vi "Package Name.vi"(8 "error in (no error)":errorcluster, 11 "InitAction in":refnum<class "InitAction.lvclass">) -> (0 "error out":errorcluster, 2 "Package Name":string, 3 "InitAction out":refnum<class "InitAction.lvclass">)   [LabVIEW 2020, in "GPackTools.lvlib" / "InitAction.lvclass"]
uses:
  InitAction.lvclass
  InitAction.lvclass/InitAction.ctl
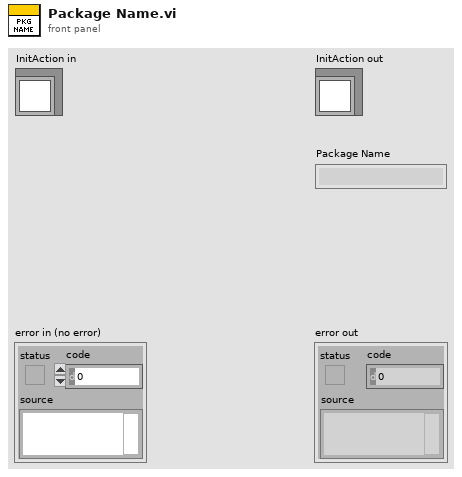
[diagram p1: front panel]
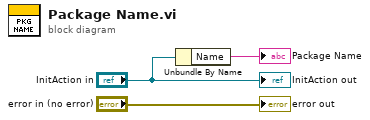
[diagram p0: block diagram]
diagram:
  n1 = Unbundle By Name("InitAction in") -> ("Name"=→"Package Name":string)
  "error out" <- "error in (no error)"
  "InitAction out" <- "InitAction in"
